vi "PRAT Sequence Description.vi"(8 "Error In":errorcluster, 11 "Test Seq":T1[](array[typedef])=[{"Sequence #"=1.0, "Cycles"=4, "Mode Setting"="", "Flow Rate (GPM)"=0.0, "Temperature (F)"=0.0, "Reset Timer"=FALSE, "Use Temp Decline Method"=FALSE, "Terminate Condition"=enum."C1-Terminate Draw @ Gallon Mark", "Condition Value #1"=0.0, "UE"=FALSE, "LE"=FALSE, "Comp"=FALSE, "Fan"=FALSE, "Test End Time (Sec)"=0.0, "Purge Until Cutout"=FALSE, "Start Conditions"=enum."Heat Source Cutout", "Condition Value #2"=0.0, "Remove Power"=FALSE, "Time"=0.0, "Check Special Cond."=enum."SC2-Check Heat Source (On-C2/Off-C1)", "Condition#"=enum."C1", "Draw Flags"=enum."N/A", "Data Processing Delay (FHD 15sec, UEF 5 Sec)"=0.0, "Test Complete"=FALSE}, {"Sequence #"=2.0, "Cycles"=9, "Mode Setting"="", "Flow Rate (GPM)"=0.0, "Temperature (F)"=0.0, "Reset Timer"=FALSE, "Use Temp Decline Method"=FALSE, "Terminate Condition"=enum."C1-Terminate Draw @ Gallon Mark", "Condition Value #1"=0.0, "UE"=FALSE, "LE"=FALSE, "Comp"=FALSE, "Fan"=FALSE, "Test End Time (Sec)"=0.0, "Purge Until Cutout"=FALSE, "Start Conditions"=enum."Heat Source Cutout", "Condition Value #2"=0.0, "Remove Power"=FALSE, "Time"=0.0, "Check Special Cond."=enum."SC2-Check Heat Source (On-C2/Off-C1)", "Condition#"=enum."C1", "Draw Flags"=enum."N/A", "Data Processing Delay (FHD 15sec, UEF 5 Sec)"=0.0, "Test Complete"=FALSE}, {"Sequence #"=3.0, "Cycles"=2, "Mode Setting"="", "Flow Rate (GPM)"=0.0, "Temperature (F)"=0.0, "Reset Timer"=FALSE, "Use Temp Decline Method"=FALSE, "Terminate Condition"=enum."C1-Terminate Draw @ Gallon Mark", "Condition Value #1"=0.0, "UE"=FALSE, "LE"=FALSE, "Comp"=FALSE, "Fan"=FALSE, "Test End Time (Sec)"=0.0, "Purge Until Cutout"=FALSE, "Start Conditions"=enum."Heat Source Cutout", "Condition Value #2"=0.0, "Remove Power"=FALSE, "Time"=0.0, "Check Special Cond."=enum."SC2-Check Heat Source (On-C2/Off-C1)", "Condition#"=enum."C1", "Draw Flags"=enum."N/A", "Data Processing Delay (FHD 15sec, UEF 5 Sec)"=0.0, "Test Complete"=FALSE}, {"Sequence #"=4.0, "Cycles"=5, "Mode Setting"="", "Flow Rate (GPM)"=0.0, "Temperature (F)"=0.0, "Reset Timer"=FALSE, "Use Temp Decline Method"=FALSE, "Terminate Condition"=enum."C1-Terminate Draw @ Gallon Mark", "Condition Value #1"=0.0, "UE"=FALSE, "LE"=FALSE, "Comp"=FALSE, "Fan"=FALSE, "Test End Time (Sec)"=0.0, "Purge Until Cutout"=FALSE, "Start Conditions"=enum."Heat Source Cutout", "Condition Value #2"=0.0, "Remove Power"=FALSE, "Time"=0.0, "Check Special Cond."=enum."SC2-Check Heat Source (On-C2/Off-C1)", "Condition#"=enum."C1", "Draw Flags"=enum."N/A", "Data Processing Delay (FHD 15sec, UEF 5 Sec)"=0.0, "Test Complete"=FALSE}, {"Sequence #"=5.0, "Cycles"=2, "Mode Setting"="", "Flow Rate (GPM)"=0.0, "Temperature (F)"=0.0, "Reset Timer"=FALSE, "Use Temp Decline Method"=FALSE, "Terminate Condition"=enum."C1-Terminate Draw @ Gallon Mark", "Condition Value #1"=0.0, "UE"=FALSE, "LE"=FALSE, "Comp"=FALSE, "Fan"=FALSE, "Test End Time (Sec)"=0.0, "Purge Until Cutout"=FALSE, "Start Conditions"=enum."Heat Source Cutout", "Condition Value #2"=0.0, "Remove Power"=FALSE, "Time"=0.0, "Check Special Cond."=enum."SC2-Check Heat Source (On-C2/Off-C1)", "Condition#"=enum."C1", "Draw Flags"=enum."N/A", "Data Processing Delay (FHD 15sec, UEF 5 Sec)"=0.0, "Test Complete"=FALSE}, {"Sequence #"=6.0, "Cycles"=5, "Mode Setting"="", "Flow Rate (GPM)"=0.0, "Temperature (F)"=0.0, "Reset Timer"=FALSE, "Use Temp Decline Method"=FALSE, "Terminate Condition"=enum."C1-Terminate Draw @ Gallon Mark", "Condition Value #1"=0.0, "UE"=FALSE, "LE"=FALSE, "Comp"=FALSE, "Fan"=FALSE, "Test End Time (Sec)"=0.0, "Purge Until Cutout"=FALSE, "Start Conditions"=enum."Heat Source Cutout", "Condition Value #2"=0.0, "Remove Power"=FALSE, "Time"=0.0, "Check Special Cond."=enum."SC2-Check Heat Source (On-C2/Off-C1)", "Condition#"=enum."C1", "Draw Flags"=enum."N/A", "Data Processing Delay (FHD 15sec, UEF 5 Sec)"=0.0, "Test Complete"=FALSE}, {"Sequence #"=7.0, "Cycles"=2, "Mode Setting"="", "Flow Rate (GPM)"=0.0, "Temperature (F)"=0.0, "Reset Timer"=FALSE, "Use Temp Decline Method"=FALSE, "Terminate Condition"=enum."C1-Terminate Draw @ Gallon Mark", "Condition Value #1"=0.0, "UE"=FALSE, "LE"=FALSE, "Comp"=FALSE, "Fan"=FALSE, "Test End Time (Sec)"=0.0, "Purge Until Cutout"=FALSE, "Start Conditions"=enum."Heat Source Cutout", "Condition Value #2"=0.0, "Remove Power"=FALSE, "Time"=0.0, "Check Special Cond."=enum."SC2-Check Heat Source (On-C2/Off-C1)", "Condition#"=enum."C1", "Draw Flags"=enum."N/A", "Data Processing Delay (FHD 15sec, UEF 5 Sec)"=0.0, "Test Complete"=FALSE}, {"Sequence #"=8.0, "Cycles"=5, "Mode Setting"="", "Flow Rate (GPM)"=0.0, "Temperature (F)"=0.0, "Reset Timer"=FALSE, "Use Temp Decline Method"=FALSE, "Terminate Condition"=enum."C1-Terminate Draw @ Gallon Mark", "Condition Value #1"=0.0, "UE"=FALSE, "LE"=FALSE, "Comp"=FALSE, "Fan"=FALSE, "Test End Time (Sec)"=0.0, "Purge Until Cutout"=FALSE, "Start Conditions"=enum."Heat Source Cutout", "Condition Value #2"=0.0, "Remove Power"=FALSE, "Time"=0.0, "Check Special Cond."=enum."SC2-Check Heat Source (On-C2/Off-C1)", "Condition#"=enum."C1", "Draw Flags"=enum."N/A", "Data Processing Delay (FHD 15sec, UEF 5 Sec)"=0.0, "Test Complete"=FALSE}] {"Time" format="%<%H:%M:%S>t"}) -> (0 "Error Out":errorcluster, 2 "Finish Draw Count":i32[](array[numeric]), 3 "Out Description":string[](array[string]))   [LabVIEW 2016]
uses:
  Type Definitions/PRAT Test.ctl
  Utility/Save File/File Setup (Public)/Type Definition/Save File HEWH Heating Control Mode.ctl
  Draw Water Specific/Type Definitions/Terminate Draw Conditions.ctl
  Type Definitions/HEWH Start Conditions.ctl
  Draw Water Specific/Type Definitions/Check Special Condtions.ctl
  Draw Water Specific/Type Definitions/HEWH Special Condition Check.ctl
  Type Definitions/HEWH Draw Flag ENUM.ctl
  Utility/Save File/File Setup.lvlib
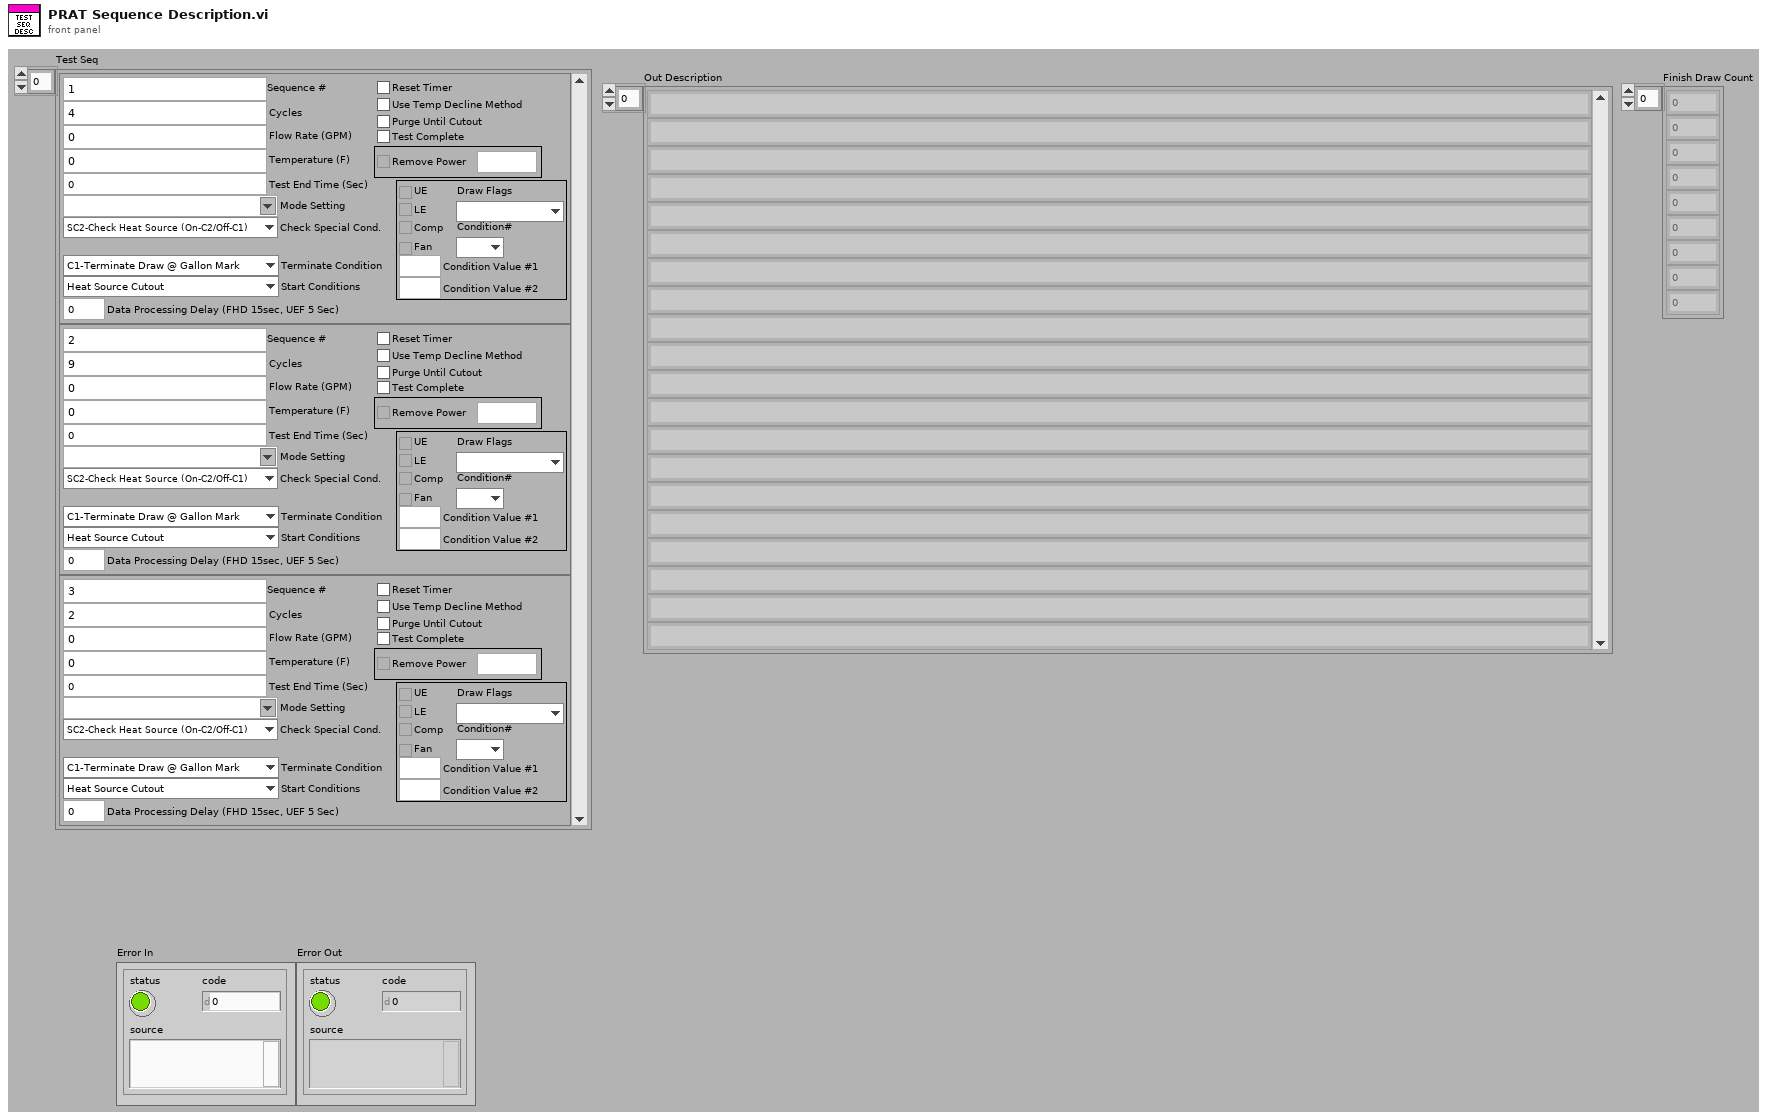
[diagram p1: front panel]
types:
  T1 = typedef "PRAT Test.ctl" = cluster{"Sequence #":dbl, "Cycles":i32, "Mode Setting":T2, "Flow Rate (GPM)":dbl, "Temperature (F)":dbl, "Reset Timer":bool, "Use Temp Decline Method":bool, "Terminate Condition":T3, "Condition Value #1":dbl, "UE":bool, "LE":bool, "Comp":bool, "Fan":bool, "Test End Time (Sec)":dbl, "Purge Until Cutout":bool, "Start Conditions":T4, "Condition Value #2":dbl, "Remove Power":bool, "Time":dbl, "Check Special Cond.":T5, "Condition#":T6, "Draw Flags":T7, "Data Processing Delay (FHD 15sec, UEF 5 Sec)":dbl, "Test Complete":bool}
  T2 = typedef "File Setup.lvlib/Save File HEWH Heating Control Mode.ctl" = string
  T3 = typedef "Terminate Draw Conditions.ctl" = enum16{"C1-Terminate Draw @ Gallon Mark", "C2-Special Last Draw (HU Test)", "C3-RTD Out <=", "C4-Mean Tank Temp <=", "C5-Decrease RTD Out (Deg F)", "C6-Time (Seconds)", "C7-Until Any Heat Source", "C8-Specific Heat Source", "C9-Do Nothing"}
  T4 = typedef "HEWH Start Conditions.ctl" = enum16{"Heat Source Cutout", "At Time (Seconds)", "Every X (Seconds)", "T2 >= X° Below Setpoint", "Seconds From Complete", "Wait for LE & Comp Cutout", "Wait for Comp Cutout", "Wait for LE Cutout", "Wait for UE Cutout"}
  T5 = typedef "Check Special Condtions.ctl" = enum16{"SC1-Do Nothing", "SC2-Check Heat Source (On-C2/Off-C1)", "SC3-Check Skip Condition", "SC4-Check Heat Source ON/Fail"}
  T6 = typedef "HEWH Special Condition Check.ctl" = enum16{"N/A", "C1", "C2", "Reset/Fail", "Skip Draw Sequence"}
  T7 = typedef "HEWH Draw Flag ENUM.ctl" = enum16{"N/A", "None(0)", "Sml(1)", "Med(2)", "SmlMed(3)", "Lrg(4)", "SmlLrg(5)", "MedLrg(6)", "SmlMedLrg(7)"}
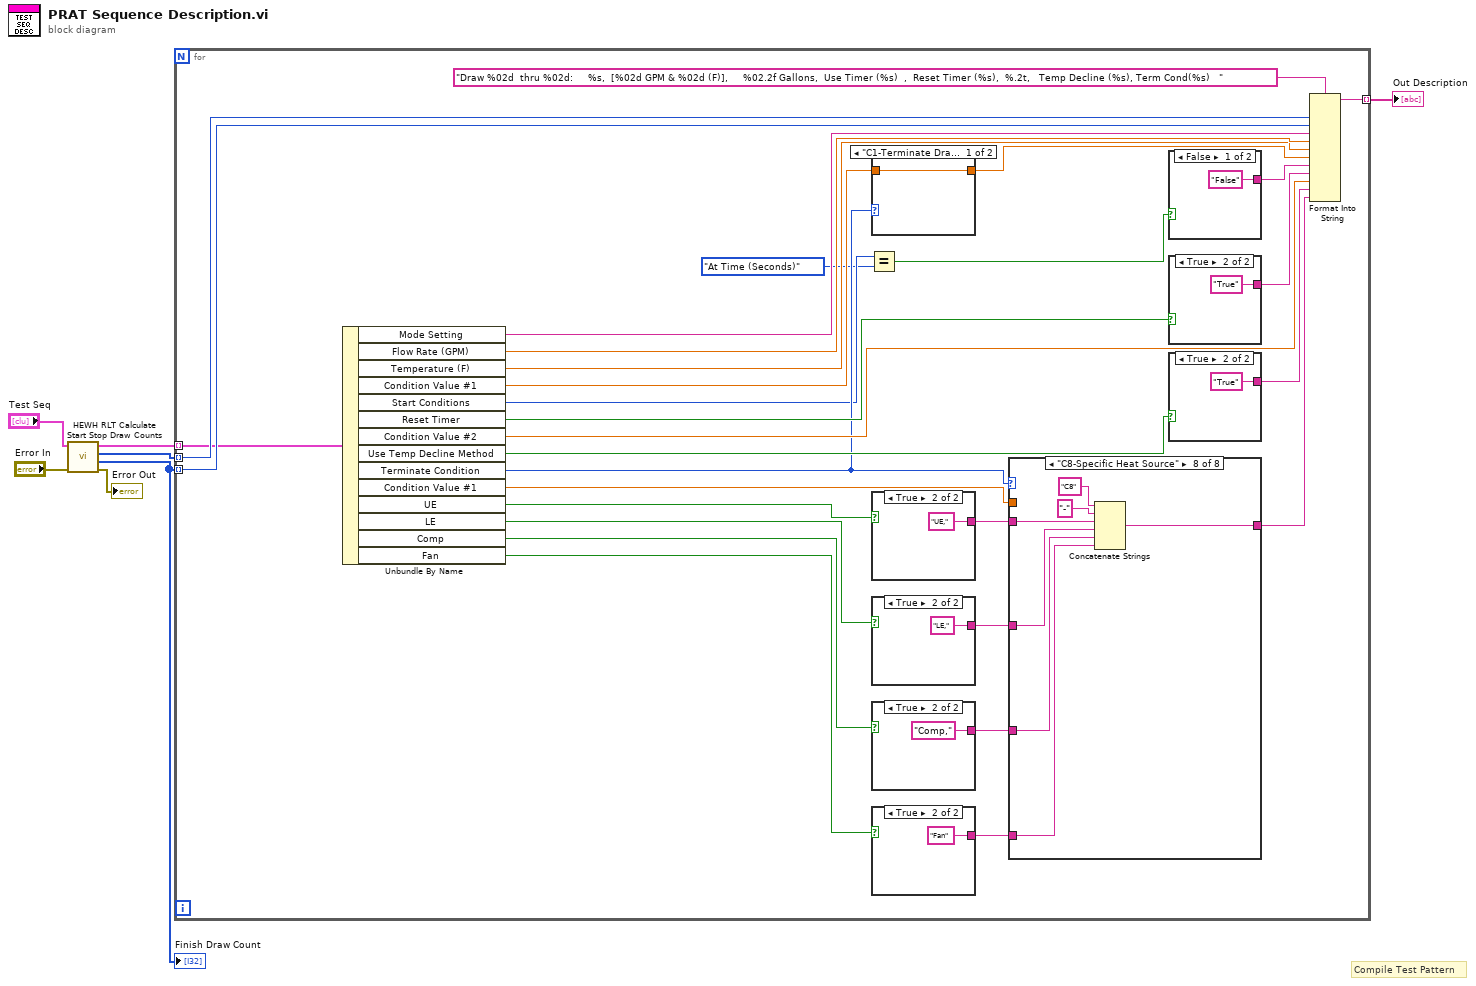
[diagram p0: block diagram]
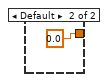
[diagram p2: hidden frame]
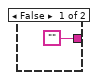
[diagram p3: hidden frame]
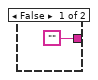
[diagram p4: hidden frame]
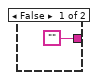
[diagram p5: hidden frame]
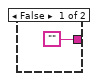
[diagram p6: hidden frame]
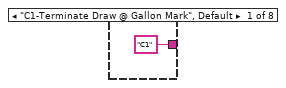
[diagram p7: hidden frame]
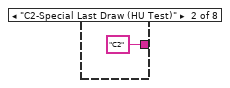
[diagram p8: hidden frame]
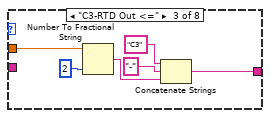
[diagram p9: hidden frame]
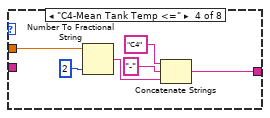
[diagram p10: hidden frame]
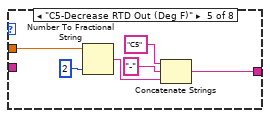
[diagram p11: hidden frame]
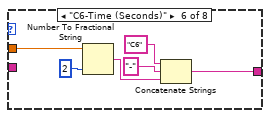
[diagram p12: hidden frame]
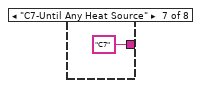
[diagram p13: hidden frame]
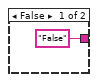
[diagram p14: hidden frame]
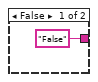
[diagram p15: hidden frame]
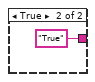
[diagram p16: hidden frame]
diagram:
  # "Compile Test Pattern"
  n1 = call "HEWH RLT Calculate Start Stop Draw Counts.vi"("Error In"="Error In", "Test Sequence In"="Test Seq") -> ("Error Out"=→"Error Out":errorcluster, "Finish Draw Count"=w4:i32[], "Start Draw Count"=w5:i32[], "Test Sequence Out"=w3:T1[])  [unwired: 6 in]
  "Finish Draw Count" <- w4
  n2 = for {
    tunnel: w5 -> [w37] mode=indexing
    tunnel: w4 -> [w36] mode=indexing
    tunnel: [w35] -> w7 mode=indexing
    tunnel: w3 -> [w33] mode=indexing
    n3 = Unbundle By Name(w33) -> ("Mode Setting"=w32:T2, "Flow Rate (GPM)"=w31:dbl, "Temperature (F)"=w30:dbl, "Condition Value #1"=w12:dbl, "Start Conditions"=w10:T4, "Reset Timer"=w27:bool, "Condition Value #2"=w29:dbl, "Use Temp Decline Method"=w25:bool, "Terminate Condition"=w13:T3, "Condition Value #1"=w22:dbl, "UE"=w21:bool, "LE"=w20:bool, "Comp"=w19:bool, "Fan"=w18:bool)
    n4 = Equal?(x=w10, y=HEWH_Start_Conditions."At Time (Seconds)") -> (x = y?=w8:bool)
    n5 = case shown="\"C1-Terminate Draw @ Gallon Mark\"" w13 {
      tunnel: w12 -> [w38 _]
      tunnel: [w38 0.0 ("Condition Value")] -> w11
      frame "C1-Terminate Draw @ Gallon Mark" {
      }
      frame Default {
      }
    }
    n6 = case shown="True" w21 {
      tunnel: ["" "UE,"] -> w17
      frame False {
      }
      frame True {
      }
    }
    n7 = case shown="True" w20 {
      tunnel: ["" "LE,"] -> w16
      frame False {
      }
      frame True {
      }
    }
    n8 = case shown="True" w19 {
      tunnel: ["" "Comp,"] -> w15
      frame False {
      }
      frame True {
      }
    }
    n9 = case shown="True" w18 {
      tunnel: ["" "Fan"] -> w14
      frame False {
      }
      frame True {
      }
    }
    n10 = case shown="\"C8-Specific Heat Source\"" w13 {
      tunnel: ["C1" "C2" w50 w56 w62 w68 "C7" w75] -> w23
      tunnel: w22 -> [_ _ w51 w57 w63 w69 _ _]
      tunnel: w17 -> [_ _ _ _ _ _ _ w79]
      tunnel: w16 -> [_ _ _ _ _ _ _ w78]
      tunnel: w15 -> [_ _ _ _ _ _ _ w77]
      tunnel: w14 -> [_ _ _ _ _ _ _ w76]
      frame "C1-Terminate Draw @ Gallon Mark", Default {
      }
      frame "C2-Special Last Draw (HU Test)" {
      }
      frame "C3-RTD Out <=" {
        n11 = Number To Fractional String(number=w51, precision (6)=i16 2) -> (F-format string=w55:string)  [unwired: 2 in]
        n12 = Concatenate Strings("C3", "-" ("string"), w55) -> (w50:string)
      }
      frame "C4-Mean Tank Temp <=" {
        n13 = Number To Fractional String(number=w57, precision (6)=i16 2) -> (F-format string=w61:string)  [unwired: 2 in]
        n14 = Concatenate Strings("C4", "-" ("string"), w61) -> (w56:string)
      }
      frame "C5-Decrease RTD Out (Deg F)" {
        n15 = Number To Fractional String(number=w63, precision (6)=i16 2) -> (F-format string=w67:string)  [unwired: 2 in]
        n16 = Concatenate Strings("C5", "-" ("string"), w67) -> (w62:string)
      }
      frame "C6-Time (Seconds)" {
        n17 = Number To Fractional String(number=w69, precision (6)=i16 2) -> (F-format string=w73:string)  [unwired: 2 in]
        n18 = Concatenate Strings("C6", "-" ("string"), w73) -> (w68:string)
      }
      frame "C7-Until Any Heat Source" {
      }
      frame "C8-Specific Heat Source" {
        n19 = Concatenate Strings("C8", "-" ("string"), w79, w78, w77, w76) -> (w75:string)
      }
    }
    n20 = case shown="False" w8 {
      tunnel: ["False" "True"] -> w28
      frame False {
      }
      frame True {
      }
    }
    n21 = case shown="True" w27 {
      tunnel: ["False" "True"] -> w26
      frame False {
      }
      frame True {
      }
    }
    n22 = case shown="True" w25 {
      tunnel: ["False" "True"] -> w24
      frame False {
      }
      frame True {
      }
    }
    n23 = Format Into String(format string="Draw %02d  thru %02d:     %s,  [%02d GPM & %02d (F)],     %02.2f Gallons,  Use Timer (%s)  ,  Reset Timer (%s),  %.2t,   Temp Decline (%s), Term Cond(%s)   ", w37, w36, w32, w31, w30, w11, w28, w26, w29, w24, w23) -> (resulting string=w35:string)  [unwired: 2 in, 1 out]
  }
  "Out Description" <- w7
